vi "Speed Sensitivity.vi"(11 "Input":dbl) -> (3 "Output":dbl)   [LabVIEW 2016]
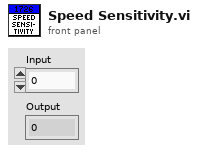
[diagram p1: front panel]
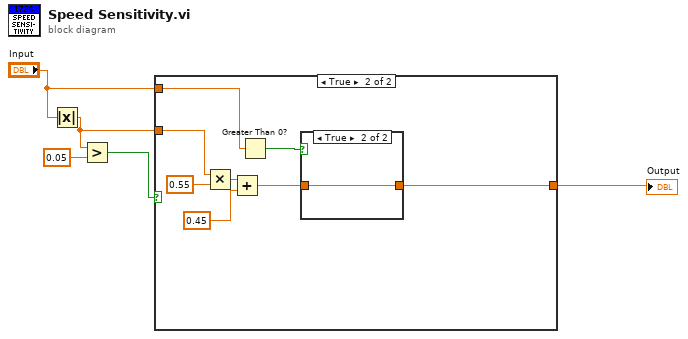
[diagram p0: block diagram]
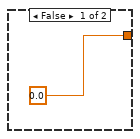
[diagram p2: hidden frame]
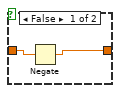
[diagram p3: hidden frame]
diagram:
  n1 = Absolute Value(x="Input") -> (abs(x)=w2:dbl)
  n2 = Greater?(x=w2, y=0.05) -> (0:w4:bool)
  n3 = case shown="True" w4 {
    tunnel: [0.0 w9] -> w3
    tunnel: w2 -> [_ w14]
    tunnel: "Input" -> [_ w7]
    frame False {
    }
    frame True {
      n4 = Multiply(x=w14, y=0.55) -> (x*y=w12:dbl)
      n5 = Add(x=w12, y=0.45) -> (x+y=w10:dbl)
      n6 = Greater Than 0?(x=w7) -> (x > 0?=w8:bool)
      n7 = case shown="True" w8 {
        tunnel: w10 -> [w16 w17]
        tunnel: [w15 w17] -> w9
        frame False {
          n8 = Negate(x=w16) -> (-x=w15:dbl)
        }
        frame True {
        }
      }
    }
  }
  "Output" <- w3
